vi "Powermeter.vi"() -> ()   [LabVIEW 2016]
uses:
  <vilib>/Utility/file.llb/Write Delimited Spreadsheet (DBL).vi
panel:
  in  "file path (dialog if empty)":path=path "C:/data/20180108/meas_after_chamber3.txt"
  out "Array":dbl[][](array[numeric])=[[7.23968355e-07, 0.000520936203831739], [1.3891347e-06, 4.000790045427755], [2.22478525e-06, 8.000538218447847], [3.17887816e-06, 12.00080732767177], [4.18567197e-06, 16.000555500691863], [5.18525303e-06, 20.000303673711954], [6.08665823e-06, 24.00057278293588], [6.81905112e-06, 28.00032095595597], [7.35101412e-06, 32.00111100138373], [7.63557455e-06, 36.00033823819999], [7.64861943e-06, 40.00112828362774], [7.39451934e-06, 44.00087645664783], [6.88487489e-06, 48.00114556587176], [6.14666351e-06, 52.00089373889185], [5.24256257e-06, 55.99751629468895], [4.25977896e-06, 60.0014319573397], [3.26209624e-06, 64.00118013035978], [2.29907482e-06, 68.0014492395837], [1.45085585e-06, 72.0011974126038], [7.881589e-07, 75.99729903219708], [3.49692584e-07, 79.997568141421], [1.51275032e-07, 83.9973163144411], [2.0445826e-07, 88.00123197709183], [5.01498675e-07, 92.00150108631576], [1.00482805e-06, 95.99708176970519], [1.66616496e-06, 100.00151836855977], [2.44069224e-06, 104.0017874777837], [3.26173131e-06, 107.99736816117314], [4.05045967e-06, 112.00128382382388], [4.73985529e-06, 116.0015529330478], [5.28320334e-06, 119.99713361643724], [5.64147467e-06, 123.99740272566116], [5.77012042e-06, 128.00131838831192], [5.66463677e-06, 132.00158749753584], [5.341004e-06, 135.9976891171291], [4.80983363e-06, 140.00160477977985], [4.10490293e-06, 144.00187388900378], [3.31128672e-06, 147.99745457239322], [2.49440768e-06, 151.99772368161715], [1.71064312e-06, 155.99747185463724], [1.01484557e-06, 159.99722002765733], [4.86414649e-07, 164.00217756271573], [1.6947682e-07, 167.99723730990135], [9.10798263e-08, 172.00167390875592], [2.64213355e-07, 175.9977755283492], [6.88614307e-07, 179.99856557377694], [1.33746948e-06, 184.00248123642768], [2.15841192e-06, 187.99702004740945], [3.09896518e-06, 191.99885196524488], [4.10840221e-06, 195.99807920206115], [5.10472228e-06, 200.00251580091572], [6.00240219e-06, 203.99809648430517], [6.74169814e-06, 208.00253308315973], [7.29747853e-06, 211.99811376654918], [7.5919761e-06, 215.99890381197693], [7.62490117e-06, 220.00281947462767], [7.38062772e-06, 223.99735828560944], [6.88778664e-06, 228.00231582066786], [6.16340549e-06, 231.99893837646496], [5.26183021e-06, 236.0028540391157], [4.28055182e-06, 239.99843472250515], [3.29009595e-06, 243.9976619593214], [2.3326154e-06, 247.99845200474917], [1.48282641e-06, 251.99820017776923], [8.06699404e-07, 256.0000320956047], [3.58600659e-07, 260.0029058858477], [1.52494025e-07, 263.9984865692372], [1.96607701e-07, 267.9987556784611], [4.85442968e-07, 271.999024787685], [9.85953989e-07, 275.9982520245013], [1.64411836e-06, 280.0032095595597], [2.41025714e-06, 283.9982693067453], [3.22702226e-06, 287.9995802883769], [4.02502474e-06, 291.99828658898934], [4.72426973e-06, 295.99907663441707], [5.27813518e-06, 299.99778293502953], [5.62844798e-06, 303.9980520442534], [5.76201955e-06, 307.9988420896812], [5.64809307e-06, 311.9991111989051], [5.3047811e-06, 315.99781749951757], [4.77325148e-06, 319.9986075449453], [4.08379856e-06, 323.9983557179654], [3.28954229e-06, 327.9986248271893], [2.46272657e-06, 331.99889393641325], [1.67599762e-06, 336.0002049180448], [9.92885361e-07, 339.99891121865727], [4.67702193e-07, 343.9976175192697], [1.58591646e-07, 347.9989285009013], [9.39398035e-08, 351.9981557377175], [2.81438361e-07, 356.0041551451836]]
  in  "step size":dbl=4.0
  in  "Start":dbl
  in  "N of steps":i32=90
  out "Power":dbl=2.81438361e-07
  in  "Wavelength (0.0)":dbl=1064.0
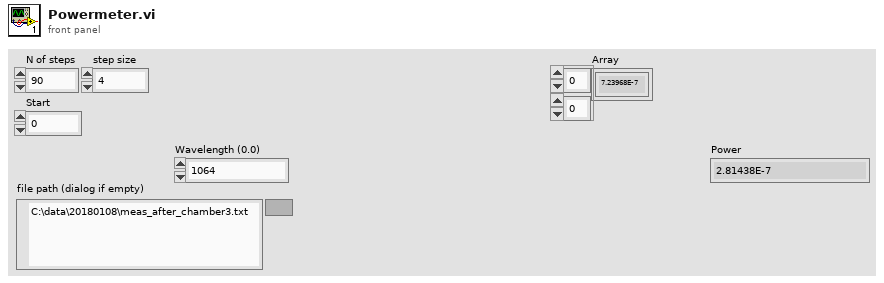
[diagram p1: front panel]
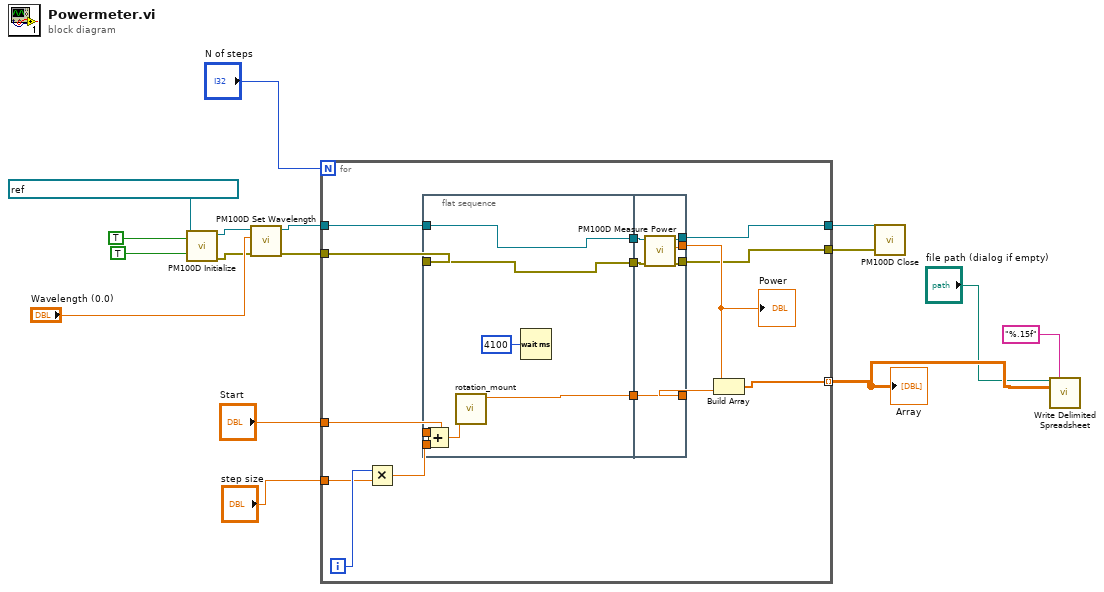
[diagram p0: block diagram]
diagram:
  n1 = call <instrlib>:"PM100D Initialize.vi"("Reset Device (Reset Device)"=TRUE, "ID Query (Do Query)"=TRUE, "resource name"=refnum<visa-resource-name> "USB0::0x1313::0x8078::P0014456::INSTR") -> ("error out"=w7:errorcluster, "instrument handle out"=w9:refnum<visa-resource-name>)  [unwired: 7 in]
  n2 = call <instrlib>:"PM100D Set Wavelength.vi"("error in (no error)"=w7, "Wavelength (0.0)"="Wavelength (0.0)", "instrument handle"=w9) -> ("error out"=w6:errorcluster, "instrument handle out"=w8:refnum<visa-resource-name>)  [unwired: 7 in]
  n3 = for {
    N: "N of steps" -> [_]
    tunnel: "Start" -> [w30]
    tunnel: "step size" -> [w28]
    tunnel: w8 -> [w24]
    tunnel: w6 -> [w23]
    tunnel: [w22] -> w5
    tunnel: [w21] -> w4
    tunnel: [w17] -> w3 mode=indexing
    i -> [w29]
    n4 = Multiply(x=w29, y=w28) -> (x*y=w27:dbl)
    n5 = flat-sequence {
      tunnel: w30 -> [w37]
      tunnel: w27 -> [w36]
      tunnel: w24 -> [w33]
      tunnel: w23 -> [w32]
      tunnel: [w34] -> w20
      tunnel: [w33] -> w19
      tunnel: [w32] -> w18
      tunnel: [w40] -> w21
      tunnel: [w39] -> w22
      tunnel: [w43] -> w25
      tunnel: [w38] -> w26
      tunnel: w20 -> [w43]
      tunnel: w19 -> [w42]
      tunnel: w18 -> [w41]
      frame #0 {
        n6 = Add(x=w37, y=w36) -> (x+y=w35:dbl)
        n7 = call "rotation_mount.vi"("position"=w35) -> ("GetPositionCounter"=w34:dbl)  [unwired: 10 in]
        n8 = Wait (ms)(milliseconds to wait=u32 4100) -> ()  [unwired: 1 out]
      }
      frame #1 {
        n9 = call <instrlib>:"PM100D Measure Power.vi"("error in (no error)"=w41, "instrument handle"=w42) -> ("error out"=w40:errorcluster, "Power"=w38:dbl, "instrument handle out"=w39:refnum<visa-resource-name>)  [unwired: 7 in]
      }
    }
    n10 = Build Array(w26, w25) -> (w17:dbl[])
    "Power" <- w26
  }
  "Array" <- w3
  n11 = call <instrlib>:"PM100D Close.vi"("error in (no error)"=w4, "instrument handle"=w5) -> ()  [unwired: 9 in, 1 out]
  n12 = call-poly <vilib>:"Write Delimited Spreadsheet.vi"("file path (dialog if empty)"="file path (dialog if empty)", "format (%.3f)"="%.15f", "2D data"=w3) -> ()  [unwired: 11 in, 2 out]
